vi "CO TCP Packet_v2.1.vi"(0 "ID":string, 5 "Version":string, 7 "TCP Packet Content":string, 9 "utc_time":u32, 11 "ue9LJ temp":u16, 13 "Data Array":string[](array[string])) -> (8 "TCP Binary Packet":string)   [LabVIEW 2014]
panel:
  out "array":string[](array[string])
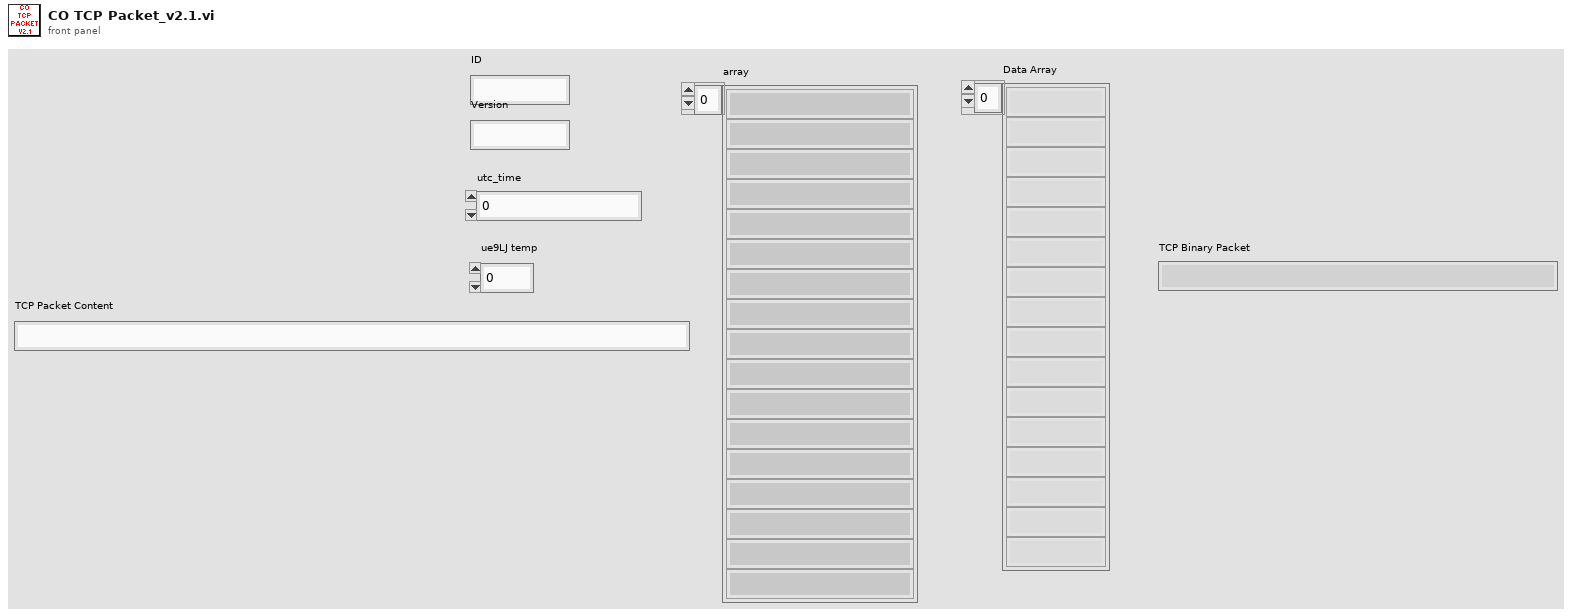
[diagram p1: front panel]
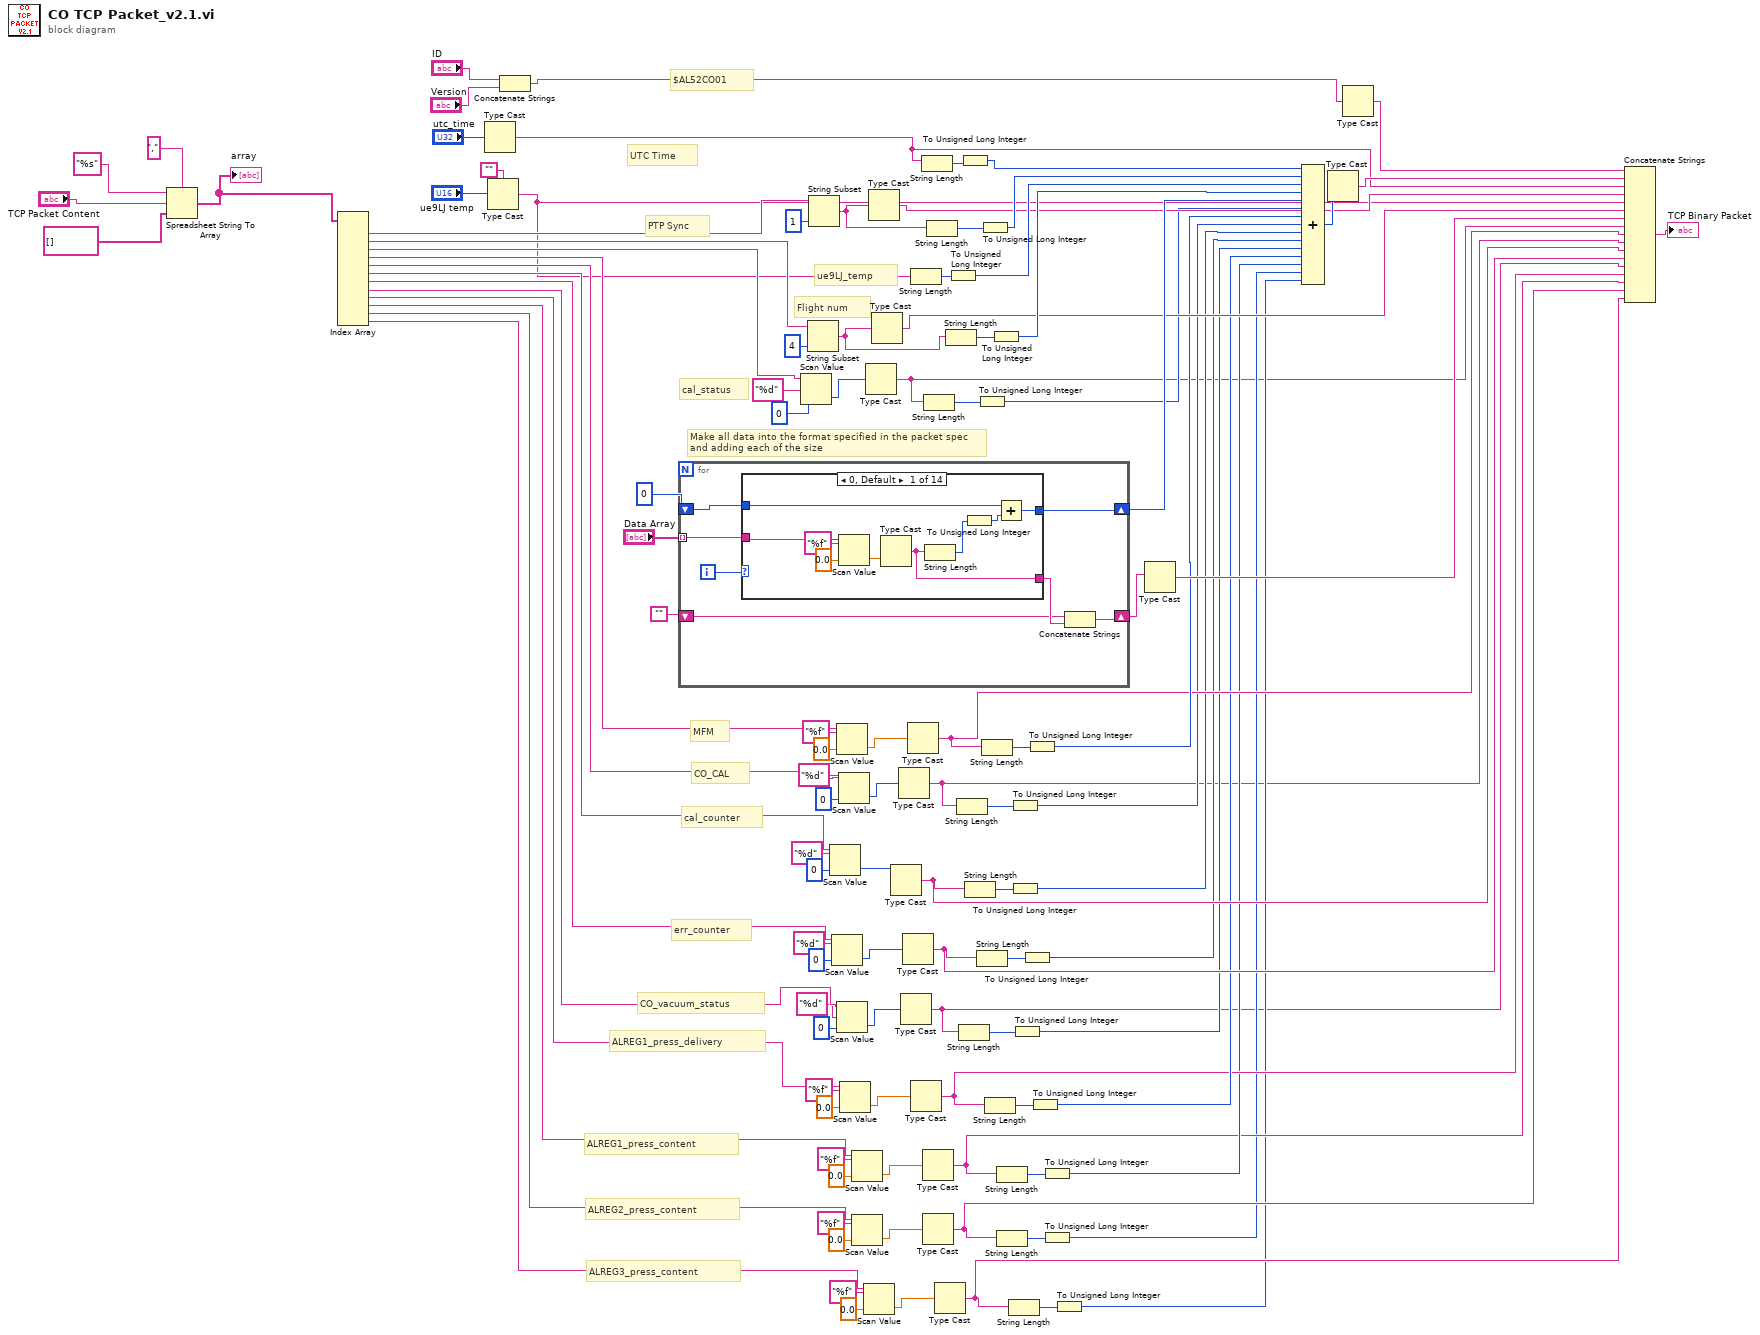
[diagram p0: block diagram]
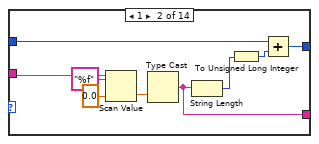
[diagram p2: hidden frame]
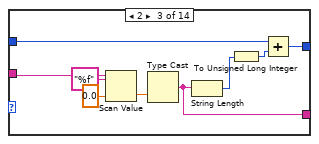
[diagram p3: hidden frame]
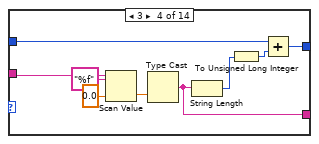
[diagram p4: hidden frame]
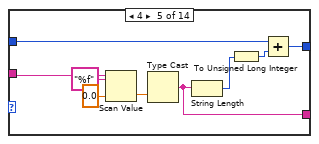
[diagram p5: hidden frame]
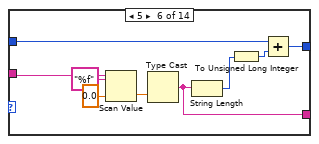
[diagram p6: hidden frame]
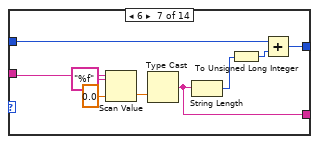
[diagram p7: hidden frame]
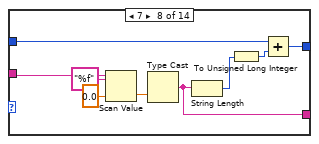
[diagram p8: hidden frame]
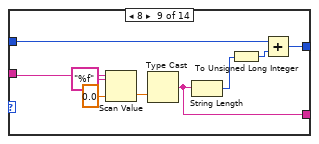
[diagram p9: hidden frame]
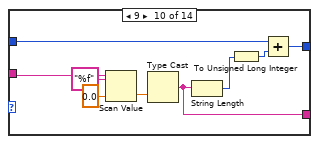
[diagram p10: hidden frame]
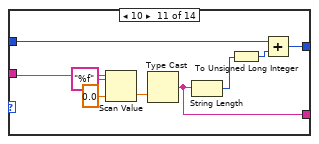
[diagram p11: hidden frame]
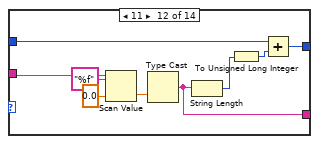
[diagram p12: hidden frame]
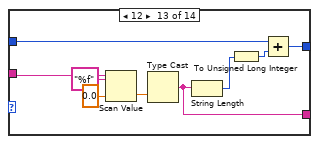
[diagram p13: hidden frame]
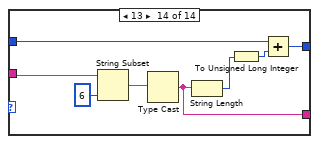
[diagram p14: hidden frame]
diagram:
  # "ALREG3_press_content"
  # "ALREG2_press_content"
  # "ALREG1_press_content"
  # "ALREG1_press_delivery"
  # "CO_vacuum_status"
  # "err_counter"
  # "cal_counter"
  # "CO_CAL"
  # "MFM"
  # "cal_status"
  # "Flight num"
  # "ue9LJ_temp"
  # "PTP Sync"
  # "UTC Time"
  # "$AL52CO01"
  # "Make all data into the format specified in the packet spec\nand adding each of the size"
  n1 = Spreadsheet String To Array(delimiter (Tab)=",", format string="%s", spreadsheet string="TCP Packet Content", array type (2D Dbl)=string[] []) -> (array=w79:string[])
  "array" <- w79
  n2 = Index Array(array=w79) -> (element #1=w4:string, element #2=w78:string, element #3=w19:string, element #4=w73:string, element #5=w24:string, element #6=w43:string, element #7=w40:string, element #8=w13:string, element #9=w36:string, element #10=w33:string, element #11=w29:string, element #12=w27:string)  [unwired: 12 in]
  n3 = Type Cast(x="utc_time") -> (*(type *) &x=w2:string)  [unwired: 1 in]
  n4 = Type Cast(type="", x="ue9LJ temp") -> (*(type *) &x=w1:string)
  n5 = Concatenate Strings("ID", "Version") -> (w3:string)
  n6 = for {
    tunnel: "Data Array" -> [w115] mode=indexing
    shift-right: [w113] -> w97
    shift-left: u32 0 -> [w114]
    shift-right: [w112] -> w86
    shift-left: "" -> [w110]
    i -> [w116]
    n7 = case shown="0, Default" w116 {
      tunnel: w115 -> [w123 w132 w141 w150 w159 w168 w177 w186 w195 w204 w213 w222 w231 w235]
      tunnel: w114 -> [w121 w130 w139 w148 w157 w166 w175 w184 w193 w202 w211 w220 w229 w241]
      tunnel: [w118 w127 w136 w145 w154 w163 w172 w181 w190 w199 w208 w217 w226 w238] -> w113
      tunnel: [w117 w126 w135 w144 w153 w162 w171 w180 w189 w198 w207 w216 w225 w237] -> w111
      frame 0, Default {
        n8 = Scan Value(string=w123, format string="%f", default (0 dbl)=sgl 0.0 ("default (0 I32)")) -> (value=w125:sgl)  [unwired: 1 out]
        n9 = Type Cast(x=w125) -> (*(type *) &x=w117:string)  [unwired: 1 in]
        n10 = String Length(string=w117) -> (length=w120:i32)
        n11 = To Unsigned Long Integer(number=w120) -> (unsigned 32bit integer=w119:u32)
        n12 = Add(x=w121, y=w119) -> (x+y=w118:u32)
      }
      frame 1 {
        n13 = Scan Value(string=w132, format string="%f", default (0 dbl)=sgl 0.0 ("default (0 I32)")) -> (value=w134:sgl)  [unwired: 1 out]
        n14 = Type Cast(x=w134) -> (*(type *) &x=w126:string)  [unwired: 1 in]
        n15 = String Length(string=w126) -> (length=w129:i32)
        n16 = To Unsigned Long Integer(number=w129) -> (unsigned 32bit integer=w128:u32)
        n17 = Add(x=w130, y=w128) -> (x+y=w127:u32)
      }
      frame 2 {
        n18 = Scan Value(string=w141, format string="%f", default (0 dbl)=sgl 0.0 ("default (0 I32)")) -> (value=w143:sgl)  [unwired: 1 out]
        n19 = Type Cast(x=w143) -> (*(type *) &x=w135:string)  [unwired: 1 in]
        n20 = String Length(string=w135) -> (length=w138:i32)
        n21 = To Unsigned Long Integer(number=w138) -> (unsigned 32bit integer=w137:u32)
        n22 = Add(x=w139, y=w137) -> (x+y=w136:u32)
      }
      frame 3 {
        n23 = Scan Value(string=w150, format string="%f", default (0 dbl)=sgl 0.0 ("default (0 I32)")) -> (value=w152:sgl)  [unwired: 1 out]
        n24 = Type Cast(x=w152) -> (*(type *) &x=w144:string)  [unwired: 1 in]
        n25 = String Length(string=w144) -> (length=w147:i32)
        n26 = To Unsigned Long Integer(number=w147) -> (unsigned 32bit integer=w146:u32)
        n27 = Add(x=w148, y=w146) -> (x+y=w145:u32)
      }
      frame 4 {
        n28 = Scan Value(string=w159, format string="%f", default (0 dbl)=sgl 0.0 ("default (0 I32)")) -> (value=w161:sgl)  [unwired: 1 out]
        n29 = Type Cast(x=w161) -> (*(type *) &x=w153:string)  [unwired: 1 in]
        n30 = String Length(string=w153) -> (length=w156:i32)
        n31 = To Unsigned Long Integer(number=w156) -> (unsigned 32bit integer=w155:u32)
        n32 = Add(x=w157, y=w155) -> (x+y=w154:u32)
      }
      frame 5 {
        n33 = Scan Value(string=w168, format string="%f", default (0 dbl)=sgl 0.0 ("default (0 I32)")) -> (value=w170:sgl)  [unwired: 1 out]
        n34 = Type Cast(x=w170) -> (*(type *) &x=w162:string)  [unwired: 1 in]
        n35 = String Length(string=w162) -> (length=w165:i32)
        n36 = To Unsigned Long Integer(number=w165) -> (unsigned 32bit integer=w164:u32)
        n37 = Add(x=w166, y=w164) -> (x+y=w163:u32)
      }
      frame 6 {
        n38 = Scan Value(string=w177, format string="%f", default (0 dbl)=sgl 0.0 ("default (0 I32)")) -> (value=w179:sgl)  [unwired: 1 out]
        n39 = Type Cast(x=w179) -> (*(type *) &x=w171:string)  [unwired: 1 in]
        n40 = String Length(string=w171) -> (length=w174:i32)
        n41 = To Unsigned Long Integer(number=w174) -> (unsigned 32bit integer=w173:u32)
        n42 = Add(x=w175, y=w173) -> (x+y=w172:u32)
      }
      frame 7 {
        n43 = Scan Value(string=w186, format string="%f", default (0 dbl)=sgl 0.0 ("default (0 I32)")) -> (value=w188:sgl)  [unwired: 1 out]
        n44 = Type Cast(x=w188) -> (*(type *) &x=w180:string)  [unwired: 1 in]
        n45 = String Length(string=w180) -> (length=w183:i32)
        n46 = To Unsigned Long Integer(number=w183) -> (unsigned 32bit integer=w182:u32)
        n47 = Add(x=w184, y=w182) -> (x+y=w181:u32)
      }
      frame 8 {
        n48 = Scan Value(string=w195, format string="%f", default (0 dbl)=sgl 0.0 ("default (0 I32)")) -> (value=w197:sgl)  [unwired: 1 out]
        n49 = Type Cast(x=w197) -> (*(type *) &x=w189:string)  [unwired: 1 in]
        n50 = String Length(string=w189) -> (length=w192:i32)
        n51 = To Unsigned Long Integer(number=w192) -> (unsigned 32bit integer=w191:u32)
        n52 = Add(x=w193, y=w191) -> (x+y=w190:u32)
      }
      frame 9 {
        n53 = Scan Value(string=w204, format string="%f", default (0 dbl)=sgl 0.0 ("default (0 I32)")) -> (value=w206:sgl)  [unwired: 1 out]
        n54 = Type Cast(x=w206) -> (*(type *) &x=w198:string)  [unwired: 1 in]
        n55 = String Length(string=w198) -> (length=w201:i32)
        n56 = To Unsigned Long Integer(number=w201) -> (unsigned 32bit integer=w200:u32)
        n57 = Add(x=w202, y=w200) -> (x+y=w199:u32)
      }
      frame 10 {
        n58 = Scan Value(string=w213, format string="%f", default (0 dbl)=sgl 0.0 ("default (0 I32)")) -> (value=w215:sgl)  [unwired: 1 out]
        n59 = Type Cast(x=w215) -> (*(type *) &x=w207:string)  [unwired: 1 in]
        n60 = String Length(string=w207) -> (length=w210:i32)
        n61 = To Unsigned Long Integer(number=w210) -> (unsigned 32bit integer=w209:u32)
        n62 = Add(x=w211, y=w209) -> (x+y=w208:u32)
      }
      frame 11 {
        n63 = Scan Value(string=w222, format string="%f", default (0 dbl)=sgl 0.0 ("default (0 I32)")) -> (value=w224:sgl)  [unwired: 1 out]
        n64 = Type Cast(x=w224) -> (*(type *) &x=w216:string)  [unwired: 1 in]
        n65 = String Length(string=w216) -> (length=w219:i32)
        n66 = To Unsigned Long Integer(number=w219) -> (unsigned 32bit integer=w218:u32)
        n67 = Add(x=w220, y=w218) -> (x+y=w217:u32)
      }
      frame 12 {
        n68 = Scan Value(string=w231, format string="%f", default (0 dbl)=sgl 0.0 ("default (0 I32)")) -> (value=w233:sgl)  [unwired: 1 out]
        n69 = Type Cast(x=w233) -> (*(type *) &x=w225:string)  [unwired: 1 in]
        n70 = String Length(string=w225) -> (length=w228:i32)
        n71 = To Unsigned Long Integer(number=w228) -> (unsigned 32bit integer=w227:u32)
        n72 = Add(x=w229, y=w227) -> (x+y=w226:u32)
      }
      frame 13 {
        n73 = String Subset(string=w235, length (rest)=6 ("length (rest)")) -> (substring=w234:string)  [unwired: 1 in]
        n74 = Type Cast(x=w234) -> (*(type *) &x=w237:string)  [unwired: 1 in]
        n75 = String Length(string=w237) -> (length=w240:i32)
        n76 = To Unsigned Long Integer(number=w240) -> (unsigned 32bit integer=w239:u32)
        n77 = Add(x=w241, y=w239) -> (x+y=w238:u32)
      }
    }
    n78 = Concatenate Strings(w110, w111) -> (w112:string)
  }
  n79 = Scan Value(string=w19, format string="%d", default (0 dbl)=u16 0) -> (value=w16:u16)  [unwired: 1 out]
  n80 = String Subset(string=w78, length (rest)=4 ("length (rest)")) -> (substring=w90:string)  [unwired: 1 in]
  n81 = String Subset(string=w4, length (rest)=1 ("length (rest)")) -> (substring=w93:string)  [unwired: 1 in]
  n82 = Scan Value(string=w43, format string="%d", default (0 dbl)=u32 0 ("default (0 I32)")) -> (value=w65:u32)  [unwired: 1 out]
  n83 = Scan Value(string=w40, format string="%d", default (0 dbl)=u32 0 ("default (0 I32)")) -> (value=w61:u32)  [unwired: 1 out]
  n84 = Scan Value(string=w73, format string="%f", default (0 dbl)=sgl 0.0 ("default (0 I32)")) -> (value=w72:sgl)  [unwired: 1 out]
  n85 = Scan Value(string=w13, format string="%d", default (0 dbl)=u16 0 ("length (rest)")) -> (value=w12:u16)  [unwired: 1 out]
  n86 = Scan Value(string=w24, format string="%d", default (0 dbl)=u16 0 ("length (rest)")) -> (value=w20:u16)  [unwired: 1 out]
  n87 = Scan Value(string=w36, format string="%f", default (0 dbl)=sgl 0.0 ("default (0 I32)")) -> (value=w56:sgl)  [unwired: 1 out]
  n88 = Scan Value(string=w33, format string="%f", default (0 dbl)=sgl 0.0 ("default (0 I32)")) -> (value=w52:sgl)  [unwired: 1 out]
  n89 = Scan Value(string=w29, format string="%f", default (0 dbl)=sgl 0.0 ("default (0 I32)")) -> (value=w48:sgl)  [unwired: 1 out]
  n90 = Scan Value(string=w27, format string="%f", default (0 dbl)=sgl 0.0 ("default (0 I32)")) -> (value=w44:sgl)  [unwired: 1 out]
  n91 = Type Cast(x=w16) -> (*(type *) &x=w15:string)  [unwired: 1 in]
  n92 = Type Cast(x=w93) -> (*(type *) &x=w92:string)  [unwired: 1 in]
  n93 = Type Cast(x=w90) -> (*(type *) &x=w91:string)  [unwired: 1 in]
  n94 = Type Cast(x=w65) -> (*(type *) &x=w41:string)  [unwired: 1 in]
  n95 = Type Cast(x=w20) -> (*(type *) &x=w21:string)  [unwired: 1 in]
  n96 = Type Cast(x=w12) -> (*(type *) &x=w11:string)  [unwired: 1 in]
  n97 = Type Cast(x=w61) -> (*(type *) &x=w38:string)  [unwired: 1 in]
  n98 = Type Cast(x=w72) -> (*(type *) &x=w71:string)  [unwired: 1 in]
  n99 = String Length(string=w1) -> (length=w104:i32)
  n100 = Type Cast(x=w56) -> (*(type *) &x=w34:string)  [unwired: 1 in]
  n101 = String Length(string=w2) -> (length=w109:i32)
  n102 = Type Cast(x=w52) -> (*(type *) &x=w31:string)  [unwired: 1 in]
  n103 = Type Cast(x=w48) -> (*(type *) &x=w30:string)  [unwired: 1 in]
  n104 = String Length(string=w15) -> (length=w85:i32)
  n105 = String Length(string=w93) -> (length=w106:i32)
  n106 = Type Cast(x=w44) -> (*(type *) &x=w26:string)  [unwired: 1 in]
  n107 = String Length(string=w90) -> (length=w101:i32)
  n108 = To Unsigned Long Integer(number=w104) -> (unsigned 32bit integer=w103:u32)
  n109 = String Length(string=w21) -> (length=w70:i32)
  n110 = String Length(string=w11) -> (length=w60:i32)
  n111 = To Unsigned Long Integer(number=w109) -> (unsigned 32bit integer=w108:u32)
  n112 = String Length(string=w41) -> (length=w68:i32)
  n113 = To Unsigned Long Integer(number=w85) -> (unsigned 32bit integer=w84:u32)
  n114 = String Length(string=w38) -> (length=w64:i32)
  n115 = To Unsigned Long Integer(number=w106) -> (unsigned 32bit integer=w105:u32)
  n116 = String Length(string=w71) -> (length=w77:i32)
  n117 = String Length(string=w34) -> (length=w59:i32)
  n118 = To Unsigned Long Integer(number=w101) -> (unsigned 32bit integer=w100:u32)
  n119 = String Length(string=w31) -> (length=w55:i32)
  n120 = String Length(string=w30) -> (length=w51:i32)
  n121 = String Length(string=w26) -> (length=w47:i32)
  n122 = To Unsigned Long Integer(number=w70) -> (unsigned 32bit integer=w69:u32)
  n123 = To Unsigned Long Integer(number=w68) -> (unsigned 32bit integer=w42:u32)
  n124 = To Unsigned Long Integer(number=w60) -> (unsigned 32bit integer=w37:u32)
  n125 = To Unsigned Long Integer(number=w64) -> (unsigned 32bit integer=w39:u32)
  n126 = To Unsigned Long Integer(number=w77) -> (unsigned 32bit integer=w76:u32)
  n127 = To Unsigned Long Integer(number=w59) -> (unsigned 32bit integer=w35:u32)
  n128 = To Unsigned Long Integer(number=w55) -> (unsigned 32bit integer=w32:u32)
  n129 = To Unsigned Long Integer(number=w51) -> (unsigned 32bit integer=w28:u32)
  n130 = To Unsigned Long Integer(number=w47) -> (unsigned 32bit integer=w25:u32)
  n131 = Type Cast(x=w86) -> (*(type *) &x=w89:string)  [unwired: 1 in]
  n132 = Compound Arithmetic op=ADD(w108, w105, w103, w100, w97, w84, w76, w69, w42, w39, w37, w35, w32, w28, w25) -> (w95:u32)
  n133 = Type Cast(x=w95) -> (*(type *) &x=w94:string)  [unwired: 1 in]
  n134 = Type Cast(x=w3) -> (*(type *) &x=w96:string)  [unwired: 1 in]
  n135 = Concatenate Strings(w96, w94, w2, w92, w1, w91, w89, w15, w71, w21, w41, w38, w11, w34, w31, w30, w26) -> (→"TCP Binary Packet":string)
